vi "Print Data Plot.vi"(5 "X-Axis":string, 6 "image data":T1, 7 "File Name":string, 8 "Comments":string) -> ()   [LabVIEW 2019]
uses:
  <vilib>/picture/picture.llb/imagedata.ctl
panel:
  out "Date":string
  out "Data Plot":picture
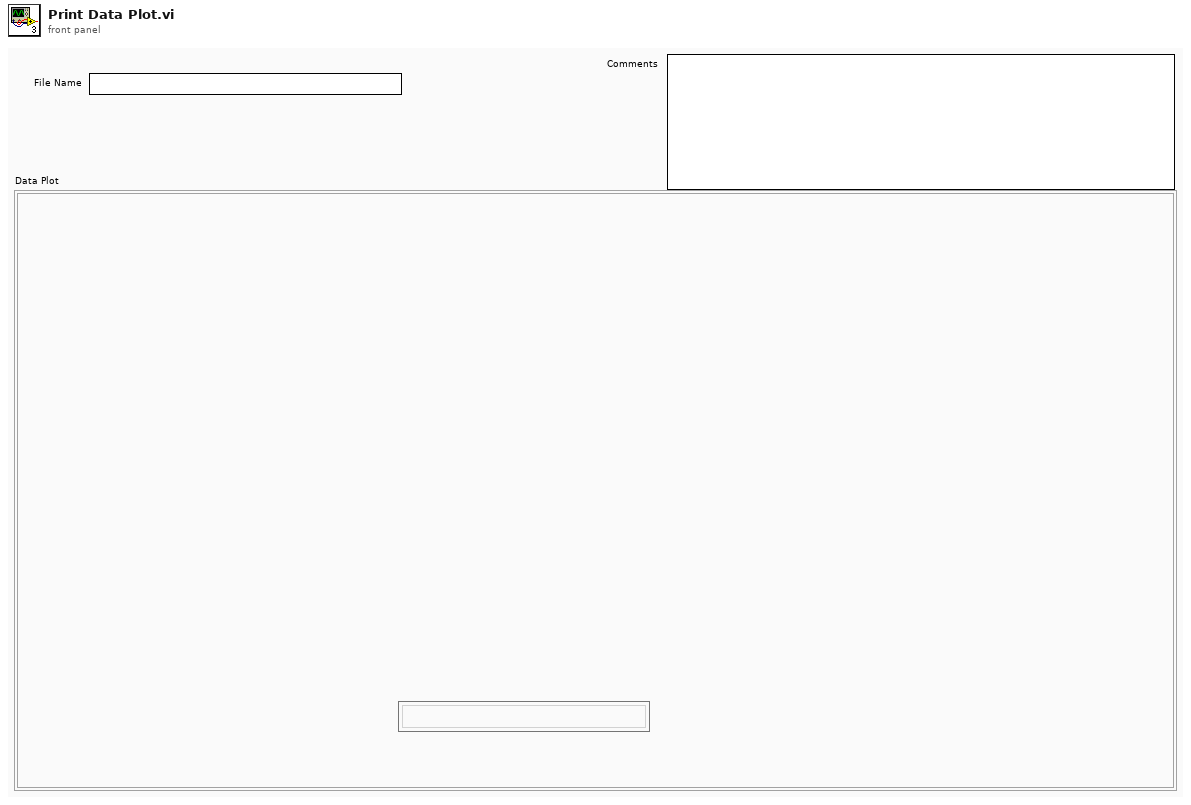
[diagram p1: front panel]
types:
  T1 = typedef "imagedata.ctl" = cluster{"image type":i32, "image depth":i32, "image":u8[], "mask":u8[], "colors":u32[], "Rectangle":cluster{"left":i16, "top":i16, "right":i16, "bottom":i16}}
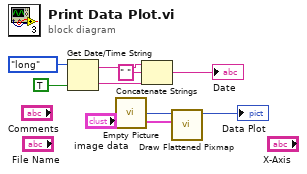
[diagram p0: block diagram]
diagram:
  n1 = Get Date/Time String(date format (0)=enum16{"short", "long", "abbreviated"}."long", want seconds? (F)=TRUE) -> (date string=w3:string, time string=w4:string)  [unwired: 1 in]
  n2 = call "Empty Picture"() -> ("empty picture"=w8:picture)
  n3 = Concatenate Strings(w3, " " ("string"), w4) -> (→"Date":string)
  n4 = call <vilib>:"Draw Flattened Pixmap.vi"("image data"="image data", "picture"=w8) -> ("new picture"=→"Data Plot":picture)  [unwired: 7 in]
